vi "main_run.vi"(4 "Runtime String":refnum<vi>, 5 "Env ready?":refnum<vi>, 6 "Cleanup?":refnum<vi>, 7 "Running?":refnum<vi>, 8 "Stop Button":refnum<vi>, 9 "Pause Button":refnum<vi>, 11 "Run":refnum<vi>) -> (2 "OK?":bool)   [LabVIEW 2019]
panel:
  # "*******************************************************************\nBiogas Plant Control\n\nAuthor: Paul Zügel\nGCSC-Frankfurt am Main 2020\n\n*******************************************************************"
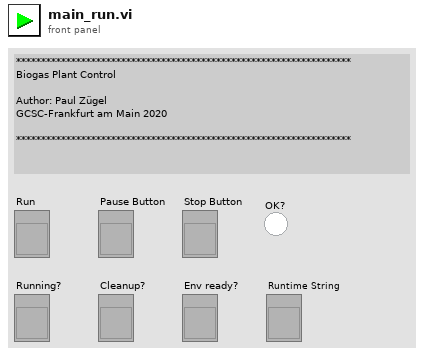
[diagram p1: front panel]
types:
  T1 = enum8{"Enabled", "Disabled", "Disabled and Grayed Out"}
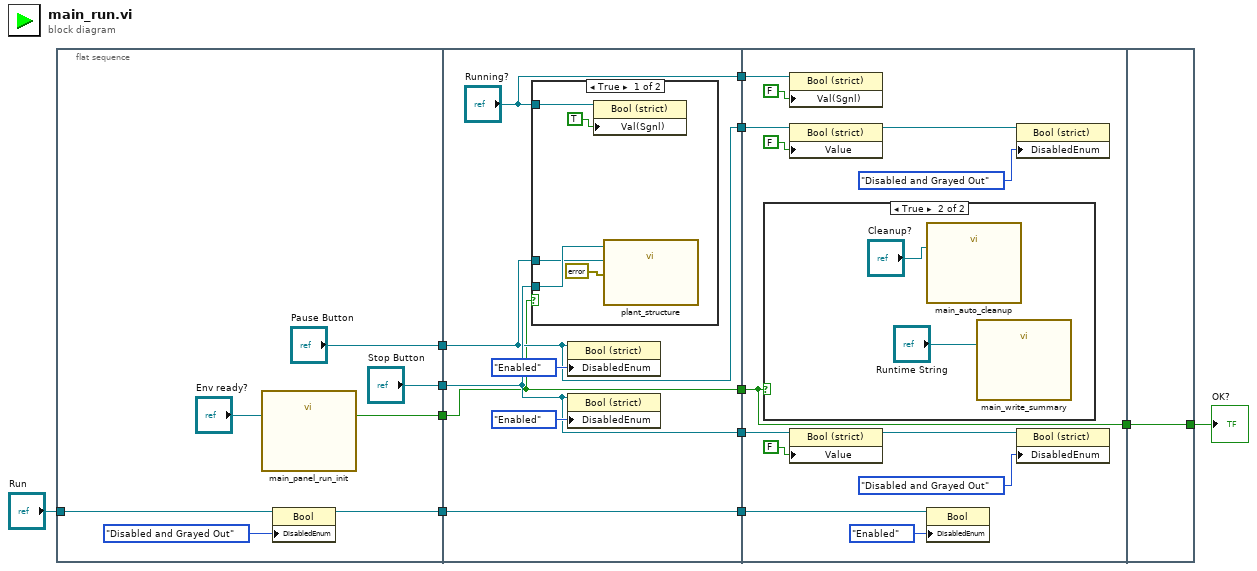
[diagram p0: block diagram]
diagram:
  n1 = flat-sequence {
    tunnel: "Run" -> [w18]
    tunnel: [w17] -> w9
    tunnel: ["Pause Button"] -> w7
    tunnel: ["Stop Button"] -> w6
    tunnel: [w14] -> w5
    tunnel: [w23] -> w12
    tunnel: [w22] -> w10
    tunnel: w9 -> [w26]
    tunnel: [w26] -> w8
    tunnel: w7 -> [w22]
    tunnel: w6 -> [w23]
    tunnel: w5 -> [w20]
    tunnel: ["Running?"] -> w4
    tunnel: [w20] -> w3
    tunnel: w12 -> [w42]
    tunnel: w10 -> [w36]
    tunnel: w8 -> [w37]
    tunnel: w4 -> [w33]
    tunnel: w3 -> [w32]
    tunnel: [w32] -> w2
    tunnel: [w47] -> w1
    tunnel: w2 -> [w47]
    frame #0 {
      n2 = call "main_panel_run_init.vi"("Env ready?"="Env ready?") -> ("OK?"=w14:bool)  [unwired: 2 in]
      n3 = property on="Property Node" class="Bool"(reference=w18, "DisabledEnum"=T1."Disabled and Grayed Out" ("Disabled")) -> (reference out=w17:refnum<vi>)  [unwired: 1 in, 1 out]
    }
    frame #1 {
      n4 = case shown="True" w20 {
        tunnel: w23 -> [w30 _]
        tunnel: w22 -> [w29 _]
        tunnel: "Running?" -> [w28 _]
        frame True {
          n5 = property on="Property Node" class="Bool (strict)"(reference=w28, "Val(Sgnl)"=TRUE ("Value (Signaling)")) -> ()  [unwired: 1 in, 2 out]
          n6 = call "plant_structure.vi"("Dataflow"=errorcluster {"status"=FALSE, "code"=0, "source"=""}, "Pause"=w29, "Stop"=w30) -> ()  [unwired: 9 in]
        }
        frame False {
        }
      }
      n7 = property on="Property Node" class="Bool (strict)"(reference=w22, "DisabledEnum"=T1."Enabled" ("Disabled")) -> ()  [unwired: 1 in, 2 out]
      n8 = property on="Property Node" class="Bool (strict)"(reference=w23, "DisabledEnum"=T1."Enabled" ("Disabled")) -> ()  [unwired: 1 in, 2 out]
    }
    frame #2 {
      n9 = case shown="True" w32 {
        frame False {
        }
        frame True {
          n10 = call "main_auto_cleanup.vi"("Cleanup?"="Cleanup?") -> ()  [unwired: 11 in]
          n11 = call "main_write_summary.vi"("Runtime String"="Runtime String") -> ()  [unwired: 11 in]
        }
      }
      n12 = property on="Property Node" class="Bool (strict)"(reference=w33, "Val(Sgnl)"=FALSE ("Value (Signaling)")) -> ()  [unwired: 1 in, 2 out]
      n13 = property on="Property Node" class="Bool (strict)"(reference=w36, "Value"=FALSE ("Stop Button")) -> (reference out=w35:refnum<vi>)  [unwired: 1 in, 1 out]
      n14 = property on="Property Node" class="Bool (strict)"(reference=w42, "Value"=FALSE) -> (reference out=w34:refnum<vi>)  [unwired: 1 in, 1 out]
      n15 = property class="Bool"(reference=w37, "DisabledEnum"=T1."Enabled" ("Disabled")) -> ()  [unwired: 1 in, 2 out]
      n16 = property class="Bool (strict)"(reference=w35, "DisabledEnum"=T1."Disabled and Grayed Out" ("Disabled")) -> ()  [unwired: 1 in, 2 out]
      n17 = property class="Bool (strict)"(reference=w34, "DisabledEnum"=T1."Disabled and Grayed Out" ("Disabled")) -> ()  [unwired: 1 in, 2 out]
    }
    frame #3 {
    }
  }
  "OK?" <- w1
